vi "Endpoint-Save Config.vi"(8 "Error In":errorcluster, 11 "Endpoint Config":T1[](array[typedef])) -> (0 "Error Out":errorcluster)   [LabVIEW 2020]
uses:
  Endpoint-Spec.ctl
  Endpoint-Modality.ctl
  Endpoint-Laterality.ctl
  <vilib>/Utility/sysdir.llb/System Directory Type.ctl
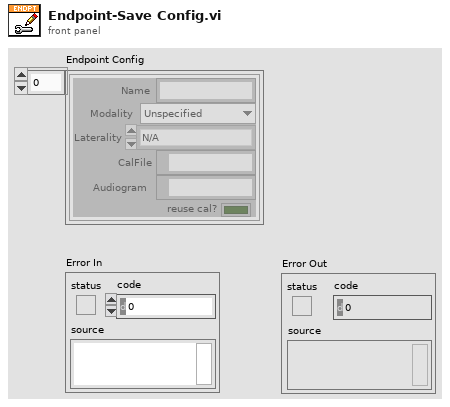
[diagram p1: front panel]
types:
  T1 = typedef "Endpoint-Spec.ctl" = cluster{"Name":string, "Modality":T2, "Laterality":T3, "CalFile":path, "Audiogram":path, "reuse cal?":bool}
  T2 = typedef "Endpoint-Modality.ctl" = enum16{"Unspecified", "Acoustic", "Electric", "Optical"}
  T3 = typedef "Endpoint-Laterality.ctl" = enum16{"N/A", "Right", "Left"}
  T4 = typedef "System Directory Type.ctl" = i32
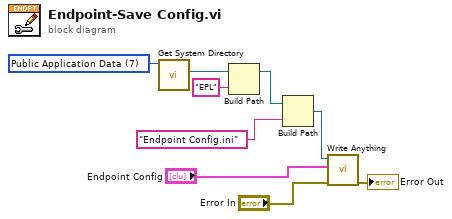
[diagram p0: block diagram]
diagram:
  w6 = T4 7 items=["User Home"=0, "User Desktop"=1, "User Documents"=2, "User Application Data"=3, "User Preferences"=4, "User Temporary"=5, "Public Documents"=6, "Public Application Data"=7, "Public Preferences"=8, "Public Cache"=13, "System Core Libraries"=9, "System Installed Libraries"=10, "Application Files"=11, "Boot Volume Root"=12] ("system directory type")
  n1 = call <vilib>:"Get System Directory.vi"("system directory type"=w6) -> ("system directory"=w5:path)  [unwired: 10 in]
  n2 = Build Path(base path=w5, name or relative path="EPL") -> (appended path=w3:path)
  n3 = Build Path(base path=w3, name or relative path="Endpoint Config.ini") -> (appended path=w1:path)
  n4 = call "Write Anything.vi"("Error In"="Error In", "Anything"="Endpoint Config", "Path (dialog)"=w1) -> ("Error Out"=→"Error Out":errorcluster)  [unwired: 7 in, 1 out]
